vi "Histogram_Setting_UI.vi"(6 "Analysis_Setting IN":T2={"PreProcess"=enum."*Algorithm*", "Parameter"=""}, 8 "error in (no error)":errorcluster, 9 "ProjectName":string, 10 "ROI List IN":refnum<vi>, 11 "Vision_Image":T7(plugin-control)) -> (0 "error out":errorcluster, 1 "Cancel?":bool, 3 "Analysis_Setting":T2={"PreProcess"=enum."*Algorithm*", "Parameter"=""})   [LabVIEW 2019]
uses:
  Controls/_UI Command Cluster/Histogram_UI Command Cluster.ctl
  <vilib>/userdefined/High Color/IMAQdx.ctl
  <vilib>/vision/NI_Vision_Development_Module.lvlib
  Controls/Analysis_Type.ctl
  Controls/Analysis_Setting.ctl
  Controls/Histogram/Analysis_Histogram_Parameter.ctl
  Controls/V_Analysis_Type.ctl
  Ctrl/VisionProcessName.ctl
panel:
  in  "Number of Classes":i32=256
  in  "Interval Range":cluster{"Minimum":sgl, "Maximum":sgl} {"Maximum" format="%.2f"; "Minimum" format="%.2f"}
  out "ROI Out":T1
  in  "Snap?":bool
  out "Numeric":i32
  in  "Done":bool
  in  "LCD_UI Command":T4(ring)
  in  "Cancel":bool
  in  "LCDTab":T5(tab)=enum."Result"
  out "Histogram Report":T6 {"Standard  Variation" format="%.2f"; "Mean Value" format="%.2f"; "Interval Width" format="%.2f"; "Starting Value" format="%.2f"; "Maximal Value" format="%.2f"; "Minimal Value" format="%.2f"}
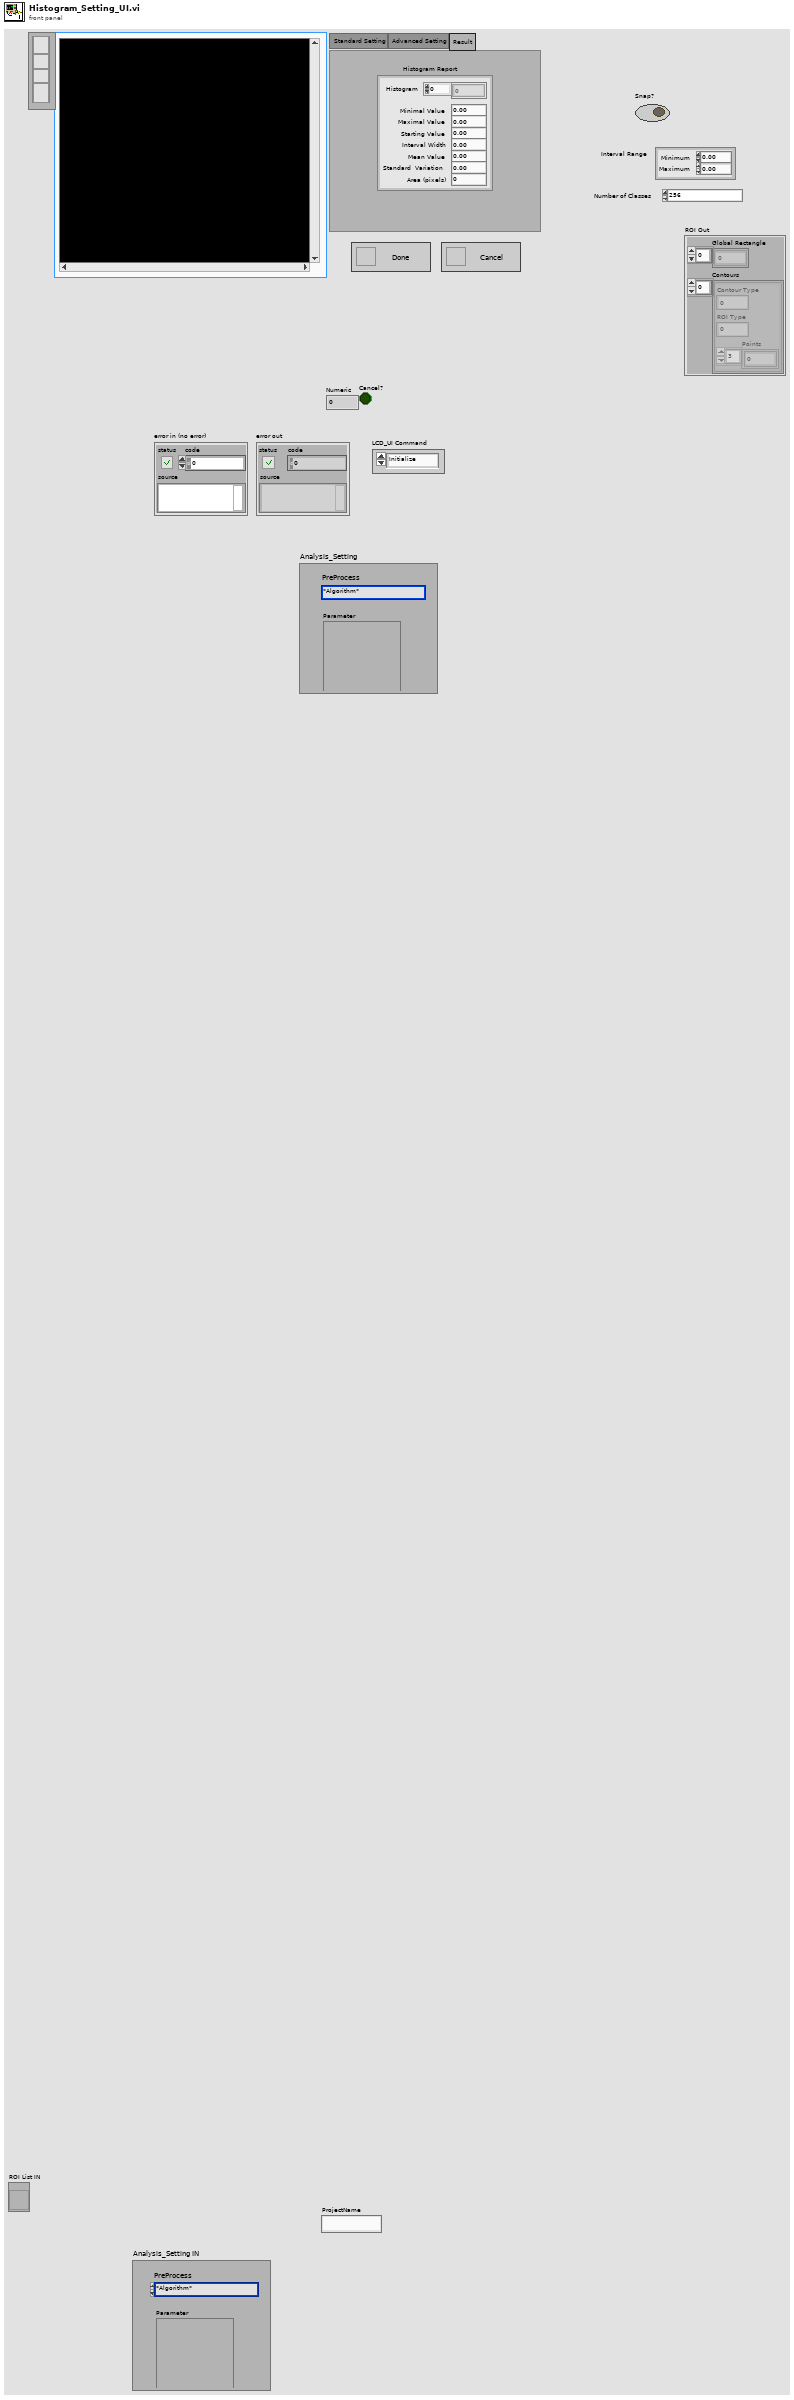
[diagram p1: front panel]
types:
  T1 = cluster{"Global Rectangle":i32[], "Contours":cluster{"Contour Type":u32, "ROI Type":u32, "Points":i32[]}[]}
  T2 = typedef "Analysis_Setting.ctl" = cluster{"PreProcess":T3, "Parameter":string}
  T3 = typedef "VisionProcessName.ctl" = enum16{"*CamParameter*", "CamAttributes", "*Preprocess*", "CG_Brightness", "C_Plane Extraction", "C_Threshold", "G_Lookup Table", "G_Threshold", "B_Image Inversion", "*Algorithm*", "CG_Histogram", "C_Color Matching", "C_Color Pattern Matching", "G_PatternMatch", "CG_Find Straight Edge", "CG_Adv. Find Straight Edge", "CG_Find Circular Edge", "G_Max Clamp", "G_Clamp (Rake)", "G_Pattern Matching"}
  T4 = enum16{"Initialize", "Done", "Run Algorithm", "Cancel"}
  T5 = enum32{"Standard Setting", "Advanced Setting", "Result"}
  T6 = cluster{"Histogram":u32[], "Minimal Value":sgl, "Maximal Value":sgl, "Starting Value":sgl, "Interval Width":sgl, "Mean Value":sgl, "Standard  Variation":sgl, "Area (pixels)":i32}
  T7 = typedef "IMAQ Image.ctl" = refnum<image>
  T8 = typedef "Histogram_UI Command Cluster.ctl" = cluster{"Histogram_UI Command":enum16{"Initialize", "Done", "Run Algorithm", "Cancel"}, "ROI":cluster{"Global Rectangle":i32[], "Contours":cluster{"Contour Type":u32, "ROI Type":u32, "Points":i32[]}[]}, "Interval Range":cluster{"Minimum":sgl, "Maximum":sgl}, "Number of Classes":i32}
  T9 = typedef "IMAQ Line" = cluster{"Start X":i32, "Start Y":i32, "End X":i32, "End Y":i32}
  T10 = typedef "IMAQdx.ctl" = refnum<k21>
  T11 = cluster{"Contour Type":u32, "ROI Type":u32, "Points":i32[]}
  T12 = typedef "Analysis_Histogram_Parameter.ctl" = cluster{"Interval Range":cluster{"Minimum":sgl, "Maximum":sgl}, "ROI Out":cluster{"Global Rectangle":i32[], "Contours":cluster{"Contour Type":u32, "ROI Type":u32, "Points":i32[]}[]}, "Number of Classes":i32}
  T13 = typedef "Analysis_Type.ctl" = u16
  T14 = typedef "Image Type" = u32
  T15 = cluster{"histogram":u32[], "Minimal Value":sgl, "Maximal Value":sgl, "Starting Value":sgl, "Interval Width":sgl, "Mean Value":sgl, "Standard  Variation":sgl, "Area (pixels)":i32}
  T16 = typedef "Analysis_Setting.ctl" = cluster{"PreProcess":T17, "Parameter":string}
  T17 = typedef "V_Analysis_Type.ctl" = enum16{"None", "C_Color Pattern Matching", "G_PatternMatching", "G_ShapeDectect", "G_GeometricMatch", "B_Area Check"}
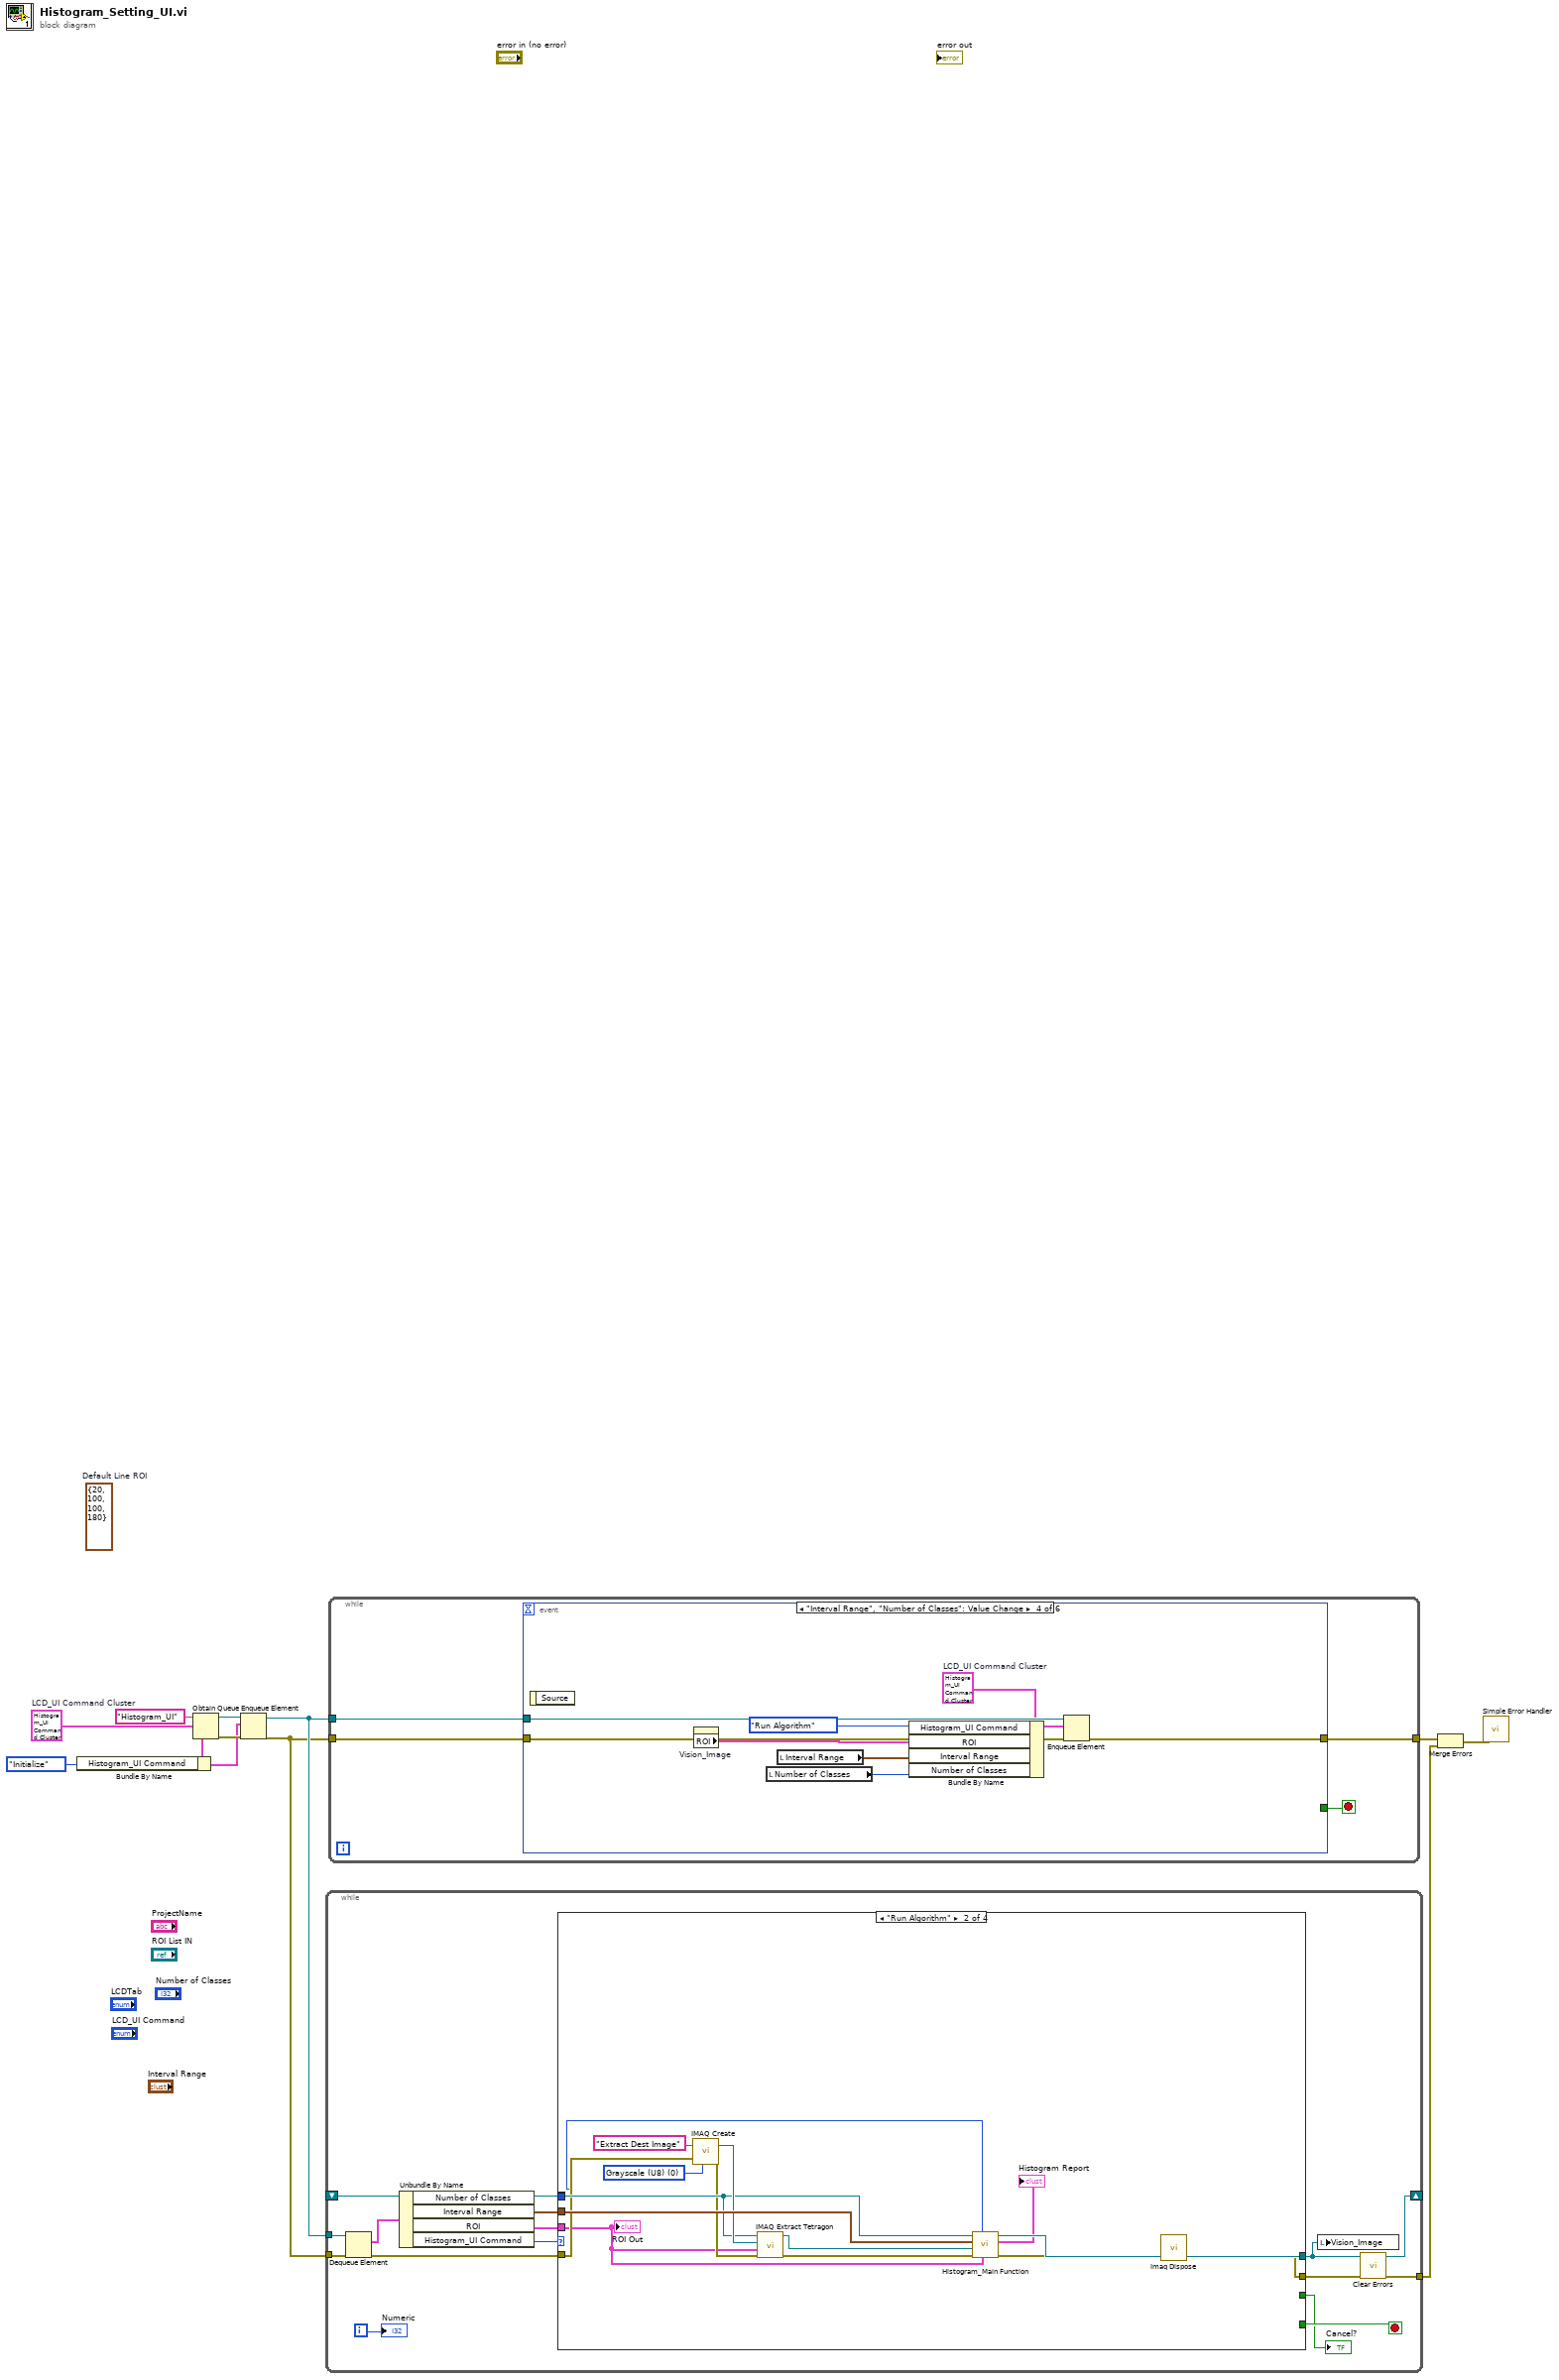
[diagram p0: block diagram]
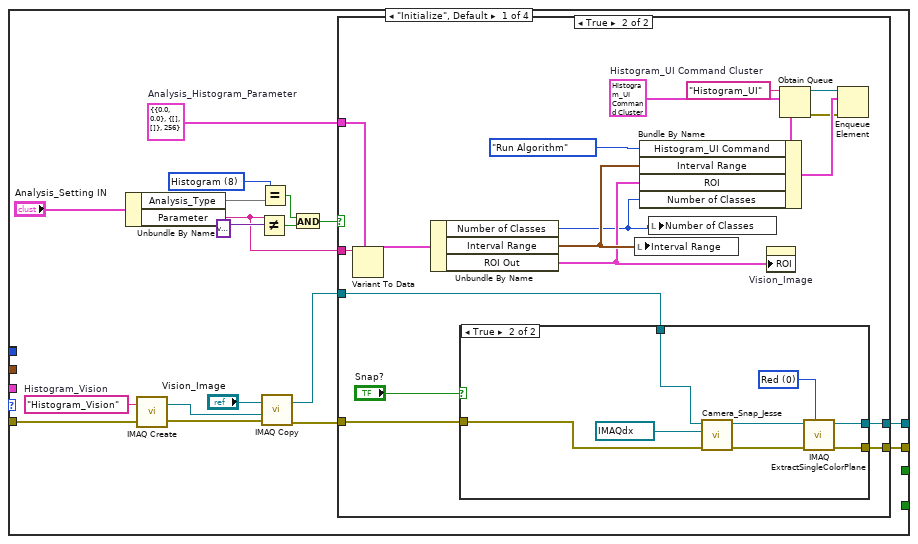
[diagram p2: hidden frame]
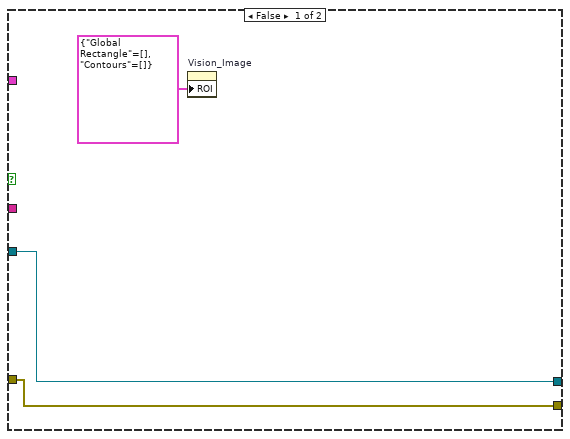
[diagram p3: hidden frame]
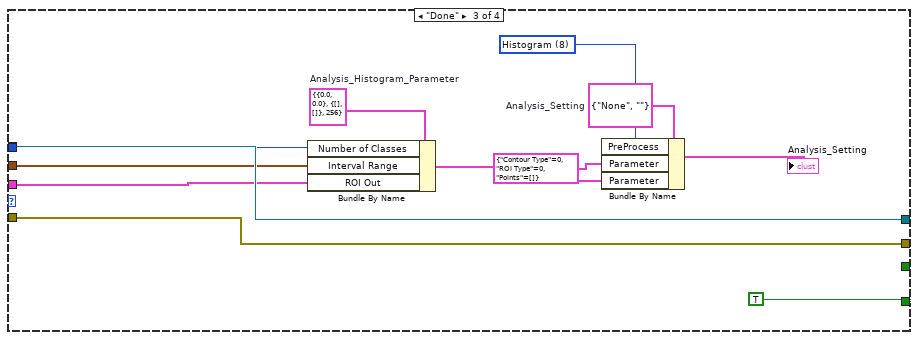
[diagram p5: hidden frame]
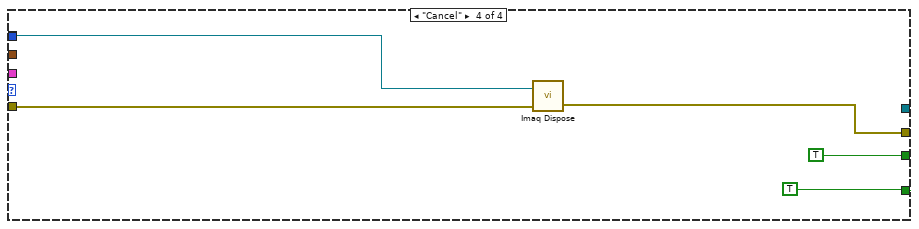
[diagram p6: hidden frame]
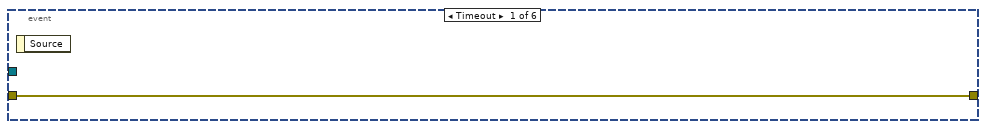
[diagram p7: hidden frame]
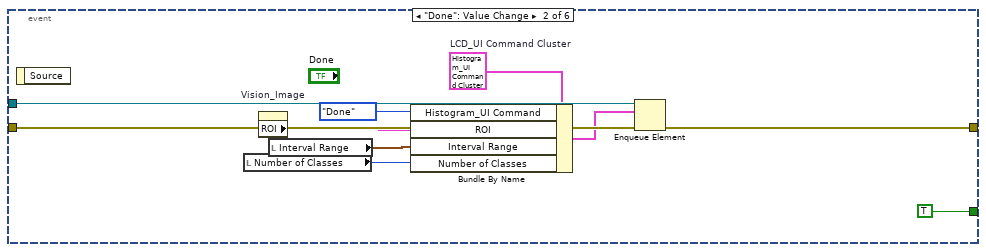
[diagram p8: hidden frame]
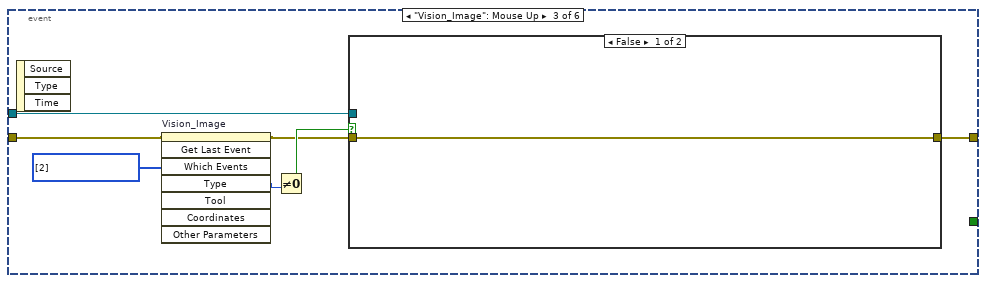
[diagram p9: hidden frame]
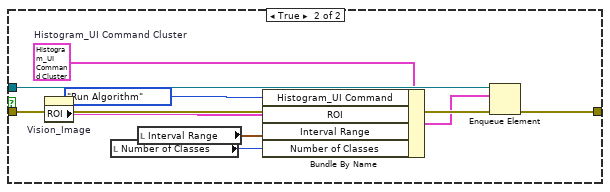
[diagram p10: hidden frame]
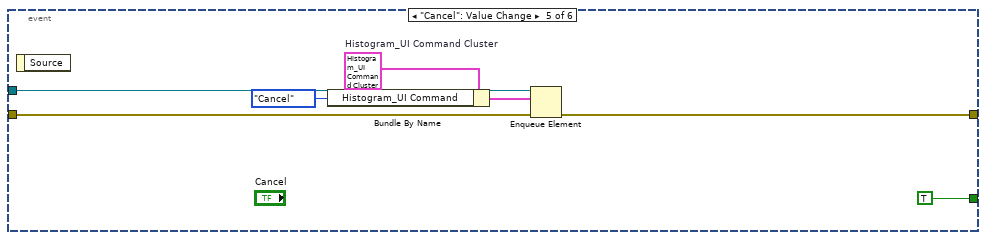
[diagram p11: hidden frame]
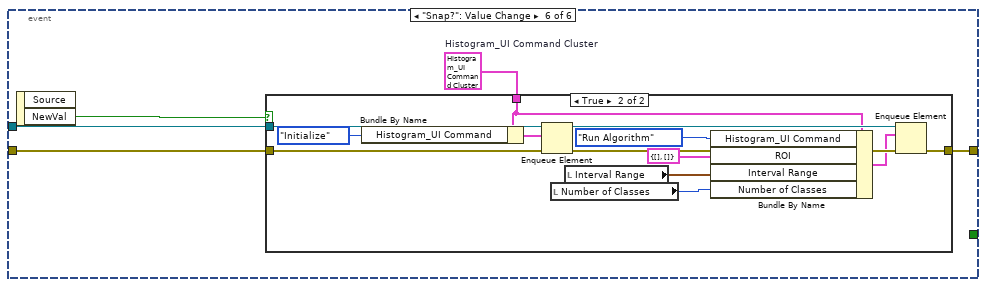
[diagram p12: hidden frame]
diagram:
  w3 = T8 {"Histogram_UI Command"=enum."Initialize", "ROI"={"Global Rectangle"=[], "Contours"=[]}, "Interval Range"={"Minimum"=1.0, "Maximum"=0.0}, "Number of Classes"=256}  # LCD_UI Command Cluster
  (unwired) T9 {"Start X"=20, "Start Y"=100, "End X"=100, "End Y"=180}  # Default Line ROI
  n1 = Bundle By Name(cluster=w3, "Histogram_UI Command"=T4."Initialize" ("Barcode 1D_UI Command")) -> (w4:T8)
  n2 = Obtain Queue(name (unnamed)="Histogram_UI", element data type=w3) -> (queue out=w11:refnum<queue>, error out=w10:errorcluster)  [unwired: 3 in, 1 out]
  n3 = Enqueue Element(queue=w11, element=w4, error in (no error)=w10) -> (queue out=w2:refnum<queue>, error out=w1:errorcluster)  [unwired: 1 in, 1 out]
  n4 = while {
    tunnel: w2 -> [w26]
    tunnel: w1 -> [w25]
    shift-right: [w16] -> _
    shift-left: _ -> [w20]
    tunnel: [w13] -> w7
    i -> [w19]
    stop <- w21 stop-if-true
    n5 = Dequeue Element(queue=w26, error in (no error)=w25) -> (element=w22:T8, error out=w23:errorcluster)  [unwired: 1 in, 2 out]
    n6 = Unbundle By Name(w22) -> ("Number of Classes"=w14:i32, "Interval Range"=w15:cluster{"Minimum":sgl, "Maximum":sgl}, "ROI"=w17:T1, "Histogram_UI Command"=w24:T4)
    n7 = case shown="\"Run Algorithm\"" w24 {
      tunnel: w23 -> [w35 w81 w99 w104]
      tunnel: [w44 w77 w99 w103] -> w12
      tunnel: [_ _ TRUE TRUE] -> w21
      tunnel: [w43 w89 w100 _] -> w16
      tunnel: w20 -> [_ w83 w100 w105]
      tunnel: [_ _ _ TRUE] -> w18
      tunnel: w17 -> [_ w75 w94 _]
      tunnel: w15 -> [_ w87 w91 _]
      tunnel: w14 -> [_ w76 w90 _]
      frame "Initialize", Default {
        w28 = T12 {"Interval Range"={"Minimum"=0.0, "Maximum"=0.0}, "ROI Out"={"Global Rectangle"=[], "Contours"=[]}, "Number of Classes"=256}  # Analysis_Histogram_Parameter
        w27 = T13 8 items=["None", "PatternMatch", "Edge Detection", "Barcode 1D", "Barcode 2D", "Clamp", "Clamp MAX", "Particle", "Histogram", "Straight Edge", "Circle", "Shape Detect", "OCR", "Contour", "ColorMatch"] ("x")
        w36 = "Histogram_Vision"  # Histogram_Vision
        n8 = Unbundle By Name("Analysis_Setting IN") -> ("Analysis_Type"=w40, "Parameter"=w29:string)
        n9 = call "IMAQ Create"("Image Name"=w36, "error in (no error)"=w35) -> ("New Image"=w33:T7, "error out"=w32:errorcluster)  [unwired: 3 in]
        n10 = Not Equal?(x=w29, y=variant) -> (x != y?=w41:bool)
        n11 = Equal?(x=w27, y=w40) -> (x = y?=w42:bool)
        n12 = call "IMAQ Copy"("error in (no error)"=w32, "Image Dst"=w33, "Image Src"="Vision_Image") -> ("error out"=w31:errorcluster, "Image Dst Out"=w30:T7)  [unwired: 3 in]
        n13 = And(x=w42, y=w41) -> (x .and. y?=w37:bool)
        n14 = case shown="True" w37 {
          tunnel: w31 -> [w46 w48]
          tunnel: [w46 w59] -> w44
          tunnel: [w47 w60] -> w43
          tunnel: w30 -> [w47 w61]
          tunnel: w29 -> [_ w64]
          tunnel: w28 -> [_ w58]
          frame False {
            n15 = property on="Vision_Image" class="ImageControl"("ROI"=T1 {"Global Rectangle"=[], "Contours"=[]}) -> ()  [unwired: 2 in, 2 out]
          }
          frame True {
            w57 = T8 {"Histogram_UI Command"=enum."Initialize", "ROI"={"Global Rectangle"=[], "Contours"=[]}, "Interval Range"={"Minimum"=1.0, "Maximum"=0.0}, "Number of Classes"=256}  # Histogram_UI Command Cluster
            n16 = Variant To Data(type=w58, Variant=w64) -> (data=w63:T12)  [unwired: 1 in, 1 out]
            n17 = Unbundle By Name(w63) -> ("Number of Classes"=w49:i32, "Interval Range"=w51:cluster{"Minimum":sgl, "Maximum":sgl}, "ROI Out"=w50:T1)
            n18 = case shown="True" "Snap?" {
              tunnel: [w66 w70] -> w59
              tunnel: [w65 w69] -> w60
              tunnel: w48 -> [w66 w67]
              tunnel: w61 -> [w65 w68]
              frame False {
              }
              frame True {
                w72 = 0 items=["Red", "Green", "Blue", "Hue", "Saturation", "Luminance", "Value", "Intensity"] ("Color Plane")
                n19 = call "Camera_Snap_Jesse.vi"("error in (no error)"=w67, "Camera Session In"=T10 "cam0", "Image In"=w68) -> ("error out"=w71:errorcluster, "New Image"=w73:T7)  [unwired: 7 in]
                n20 = call "IMAQ ExtractSingleColorPlane"("Color Plane"=w72, "error in (no error)"=w71, "Image Src"=w73) -> ("error out"=w70:errorcluster, "Image Dst Out"=w69:T7)  [unwired: 1 in, 6 out]
              }
            }
            n21 = local write "Interval Range"(w51) -> ()
            n22 = Bundle By Name(cluster=w57, "Histogram_UI Command"=T4."Run Algorithm" ("Barcode 1D_UI Command"), "Interval Range"=w51, "ROI"=w50, "Number of Classes"=w49) -> (w56:T8)
            n23 = local write "Number of Classes"(w49) -> ()
            n24 = property on="Vision_Image" class="ImageControl"("ROI"=w50) -> ()  [unwired: 2 in, 2 out]
            n25 = Obtain Queue(name (unnamed)="Histogram_UI", element data type=w57) -> (queue out=w52:refnum<queue>, error out=w53:errorcluster)  [unwired: 3 in, 1 out]
            n26 = Enqueue Element(queue=w52, element=w56, error in (no error)=w53) -> ()  [unwired: 1 in, 3 out]
          }
        }
      }
      frame "Run Algorithm" {
        w85 = T14 0 items=["Grayscale (U8)", "Grayscale (I16)", "Grayscale (SGL)", "Complex (CSG)", "RGB (U32)", "HSL (U32)", "RGB (U64)", "Grayscale (U16)"] ("Image Type")
        n27 = call "IMAQ Create"("Image Name"="Extract Dest Image", "Image Type"=w85, "error in (no error)"=w81) -> ("New Image"=w84:T7, "error out"=w80:errorcluster)  [unwired: 2 in]
        n28 = call-poly "IMAQ Extract Tetragon"("error in (no error)"=w80, "ROI Descriptor"=w75, "Image Dst"=w84, "Image Src"=w83) -> ("error out"=w79:errorcluster, "Image Dst Out"=w82:T7)  [unwired: 6 in]
        n29 = call "Histogram_Main Function.vi"("ROI Descriptor"=w75, "Number of Classes"=w76, "error in (no error)"=w79, "Image Mask"=w82, "Interval Range"=w87, "Refnum in"=w83) -> ("error out"=w78:errorcluster, "Histogram Report"=→"Histogram Report":T15, "Refnum out"=w89:T7)  [unwired: 3 in]
        n30 = call "Imaq Dispose"("error in (no error)"=w78) -> ("error out"=w77:errorcluster)  [unwired: 5 in]
        "ROI Out" <- w75
      }
      frame "Done" {
        w92 = T12 {"Interval Range"={"Minimum"=0.0, "Maximum"=0.0}, "ROI Out"={"Global Rectangle"=[], "Contours"=[]}, "Number of Classes"=256}  # Analysis_Histogram_Parameter
        w93 = T13 8 items=["None", "PatternMatch", "Edge Detection", "Barcode 1D", "Barcode 2D", "Clamp", "Clamp MAX", "Particle", "Histogram", "Straight Edge", "Circle", "Shape Detect", "OCR", "Contour", "ColorMatch"] ("Analysis_Type")
        w98 = T16 {"PreProcess"=enum."None", "Parameter"=""}  # Analysis_Setting
        n31 = Bundle By Name(cluster=w92, "Number of Classes"=w90, "Interval Range"=w91, "ROI Out"=w94) -> (w96:T12)
        n32 = Bundle By Name(cluster=w98, "PreProcess"=w93, "Parameter"=T11 {"Contour Type"=0, "ROI Type"=0, "Points"=[]} ("RegionContour"), "Parameter"=w96) -> (→"Analysis_Setting":T16)
      }
      frame "Cancel" {
        n33 = call "Imaq Dispose"("Image"=w105, "error in (no error)"=w104) -> ("error out"=w103:errorcluster)  [unwired: 4 in]
      }
    }
    "Cancel?" <- w18
    n34 = local write "Vision_Image"(w16) -> ()
    n35 = call <vilib>:"Clear Errors.vi"("error in (no error)"=w12) -> ("error out"=w13:errorcluster)  [unwired: 5 in, 1 out]
    "Numeric" <- w19
  }
  n36 = while {
    tunnel: w2 -> [w110]
    tunnel: w1 -> [w109]
    tunnel: [w107] -> w8
    stop <- w108 stop-if-true
    n37 = event shown="[3] \"Interval Range\", \"Number of Classes\": Value Change" {
      selector: _ -> [_ _ _ _ _ _]
      dyn-events: _ -> [_ _ _ _ _ _]
      timeout: _ -> [_ _ _ _ _ _]
      tunnel: w110 -> [_ w121 w128 w147 w154 w159]
      tunnel: w109 -> [w111 w120 w125 w146 w153 w158]
      tunnel: [_ TRUE _ _ TRUE _] -> w108
      tunnel: [w111 w119 w122 w145 w151 w156] -> w107
      event Timeout {
        n38 = event-data() -> ()  [unwired: 1 in, 1 out]
      }
      event "Done": Value Change {
        w118 = T8 {"Histogram_UI Command"=enum."Initialize", "ROI"={"Global Rectangle"=[], "Contours"=[]}, "Interval Range"={"Minimum"=1.0, "Maximum"=0.0}, "Number of Classes"=256}  # LCD_UI Command Cluster
        n39 = event-data() -> ()  [unwired: 1 in, 1 out]
        n40 = local read "Number of Classes"() -> (w112:i32)
        n41 = property on="Vision_Image" class="ImageControl"() -> ("ROI"=w114:T1)  [unwired: 2 in, 2 out]
        n42 = local read "Interval Range"() -> (w113:cluster{"Minimum":sgl, "Maximum":sgl})
        n43 = Bundle By Name(cluster=w118, "Histogram_UI Command"=T4."Done" ("Edge Detection_UI Command"), "ROI"=w114, "Interval Range"=w113, "Number of Classes"=w112) -> (w116:T8)
        n44 = Enqueue Element(queue=w121, element=w116, error in (no error)=w120) -> (error out=w119:errorcluster)  [unwired: 1 in, 2 out]
      }
      event "Vision_Image": Mouse Up {
        w126 = i32[] [2] items=["No Event"=0, "Click Event"=1, "Draw Event"=2, "Size Event"=4, "Scroll Event"=5, "Double Click Event"=8] ("Which Events")
        n45 = event-data() -> ()  [unwired: 1 in, 3 out]
        n46 = invoke on="Vision_Image" class="ImageControl" method="Get Last Event"(error in=w125, "Which Events"=w126) -> (error out=w124:errorcluster, "Type"=w123:i32)  [unwired: 6 in, 6 out]
        n47 = Not Equal To 0?(x=w123) -> (x != 0?=w127:bool)
        n48 = case shown="False" w127 {
          tunnel: w128 -> [_ w138]
          tunnel: w124 -> [w129 w137]
          tunnel: [w129 w134] -> w122
          frame False {
          }
          frame True {
            w132 = T8 {"Histogram_UI Command"=enum."Initialize", "ROI"={"Global Rectangle"=[], "Contours"=[]}, "Interval Range"={"Minimum"=1.0, "Maximum"=0.0}, "Number of Classes"=256}  # Histogram_UI Command Cluster
            n49 = property on="Vision_Image" class="ImageControl"() -> ("ROI"=w133:T1)  [unwired: 2 in, 2 out]
            n50 = local read "Number of Classes"() -> (w130:i32)
            n51 = local read "Interval Range"() -> (w131:cluster{"Minimum":sgl, "Maximum":sgl})
            n52 = Bundle By Name(cluster=w132, "Histogram_UI Command"=T4."Run Algorithm" ("LCD_UI Command"), "ROI"=w133, "Interval Range"=w131, "Number of Classes"=w130) -> (w135:T8)
            n53 = Enqueue Element(queue=w138, element=w135, error in (no error)=w137) -> (error out=w134:errorcluster)  [unwired: 1 in, 2 out]
          }
        }
      }
      event "Interval Range", "Number of Classes": Value Change {
        w144 = T8 {"Histogram_UI Command"=enum."Initialize", "ROI"={"Global Rectangle"=[], "Contours"=[]}, "Interval Range"={"Minimum"=1.0, "Maximum"=0.0}, "Number of Classes"=256}  # LCD_UI Command Cluster
        n54 = event-data() -> ()  [unwired: 1 in, 1 out]
        n55 = property on="Vision_Image" class="ImageControl"() -> ("ROI"=w141:T1)  [unwired: 2 in, 2 out]
        n56 = local read "Number of Classes"() -> (w139:i32)
        n57 = local read "Interval Range"() -> (w140:cluster{"Minimum":sgl, "Maximum":sgl})
        n58 = Bundle By Name(cluster=w144, "Histogram_UI Command"=T4."Run Algorithm" ("Barcode 1D_UI Command"), "ROI"=w141, "Interval Range"=w140, "Number of Classes"=w139) -> (w142:T8)
        n59 = Enqueue Element(queue=w147, element=w142, error in (no error)=w146) -> (error out=w145:errorcluster)  [unwired: 1 in, 2 out]
      }
      event "Cancel": Value Change {
        w148 = T8 {"Histogram_UI Command"=enum."Initialize", "ROI"={"Global Rectangle"=[], "Contours"=[]}, "Interval Range"={"Minimum"=1.0, "Maximum"=0.0}, "Number of Classes"=256}  # Histogram_UI Command Cluster
        n60 = event-data() -> ()  [unwired: 1 in, 1 out]
        n61 = Bundle By Name(cluster=w148, "Histogram_UI Command"=T4."Cancel" ("Barcode 1D_UI Command")) -> (w150:T8)
        n62 = Enqueue Element(queue=w154, element=w150, error in (no error)=w153) -> (error out=w151:errorcluster)  [unwired: 1 in, 2 out]
      }
      event "Snap?": Value Change {
        w155 = T8 {"Histogram_UI Command"=enum."Initialize", "ROI"={"Global Rectangle"=[], "Contours"=[]}, "Interval Range"={"Minimum"=1.0, "Maximum"=0.0}, "Number of Classes"=256}  # Histogram_UI Command Cluster
        n63 = event-data() -> ("NewVal"=w157:bool)  [unwired: 1 in, 1 out]
        n64 = case shown="True" w157 {
          tunnel: w159 -> [_ w173]
          tunnel: w158 -> [w160 w172]
          tunnel: w155 -> [_ w168]
          tunnel: [w160 w166] -> w156
          frame False {
          }
          frame True {
            n65 = Bundle By Name(cluster=w168, "Histogram_UI Command"=T4."Initialize" ("Barcode 1D_UI Command")) -> (w171:T8)
            n66 = Enqueue Element(queue=w173, element=w171, error in (no error)=w172) -> (queue out=w170:refnum<queue>, error out=w169:errorcluster)  [unwired: 1 in, 1 out]
            n67 = local read "Number of Classes"() -> (w161:i32)
            n68 = local read "Interval Range"() -> (w162:cluster{"Minimum":sgl, "Maximum":sgl})
            n69 = Bundle By Name(cluster=w168, "Histogram_UI Command"=T4."Run Algorithm" ("Barcode 1D_UI Command"), "ROI"=T1 {"Global Rectangle"=[], "Contours"=[]}, "Interval Range"=w162, "Number of Classes"=w161) -> (w167:T8)
            n70 = Enqueue Element(queue=w170, element=w167, error in (no error)=w169) -> (error out=w166:errorcluster)  [unwired: 1 in, 2 out]
          }
        }
      }
    }
  }
  n71 = Merge Errors(w8, w7) -> (w6:errorcluster)
  n72 = call <vilib>:"Simple Error Handler.vi"("error in (no error)"=w6) -> ()  [unwired: 4 in, 5 out]
